vi "Read ADC.vi"(8 "error in (no error)":errorcluster, 10 "canal":dbl, 11 "simulado in":refnum<class "simulado.lvclass">) -> (0 "error out":errorcluster, 3 "simulado out":refnum<class "simulado.lvclass">)   [LabVIEW 2019, in "simulado.lvclass"]
uses:
  simulado.lvclass
  simulado.lvclass/simulado.ctl
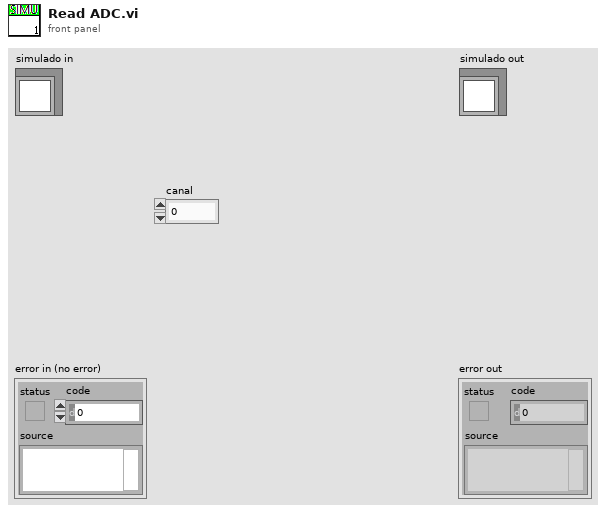
[diagram p1: front panel]
types:
  T1 = enum16{"get parameter", "Set parameters", "reset parameter", ""}
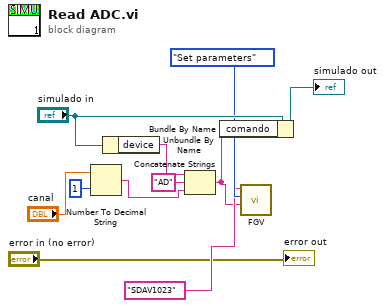
[diagram p0: block diagram]
diagram:
  n1 = Number To Decimal String(number="canal", width (-)=i16 1) -> (decimal integer string=w5:string)
  n2 = Unbundle By Name("simulado in") -> ("device"=w9:string)
  n3 = Concatenate Strings(w9, "AD" ("string"), w5) -> (w2:string)
  n4 = Bundle By Name(cluster="simulado in", "comando"=w2) -> (→"simulado out":refnum<class "simulado.lvclass">)
  n5 = call "FGV.vi"("command"=w2, "functions"=T1."Set parameters", "response to save"="SDAV1023") -> ()  [unwired: 7 in, 2 out]
  "error out" <- "error in (no error)"
